vi "RotateGH_U.vi"(2 "error in (no error)":errorcluster, 3 "controller in":refnum<k24>, 4 "U":dbl=2.0) -> (0 "error out":errorcluster, 1 "controller out":refnum<k24>)   [LabVIEW 2019]
uses:
  C:/Users/TTUHEP/Documents/LabVIEW/Other Models/2010/Bin/Aerotech.A3200.dll
  Other Models/2010/Bin/Aerotech.A3200.dll
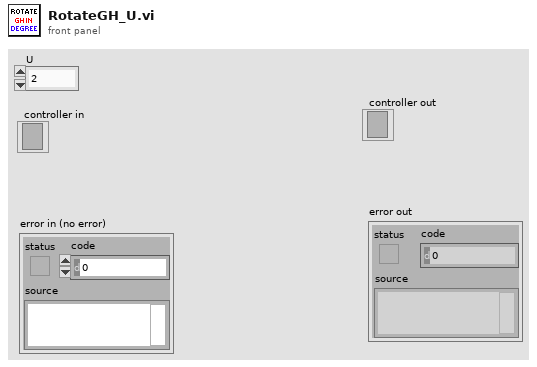
[diagram p1: front panel]
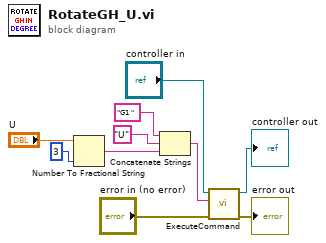
[diagram p0: block diagram]
diagram:
  n1 = Number To Fractional String(number="U", precision (6)=3) -> (F-format string=w9:string)  [unwired: 2 in]
  n2 = Concatenate Strings("G1 " ("string"), "U", w9) -> (w5:string)
  n3 = call "ExecuteCommand.vi"("error in (no error)"="error in (no error)", "Command Code"=w5, "controller in"="controller in") -> ("error out"=→"error out":errorcluster, "controller out"=→"controller out":refnum<k24>)  [unwired: 6 in, 1 out]
